vi "LVFunction_Imop_Compute_Strehl from HasoField.vi"(0 "HasoField.lvclass":refnum<class "HasoField.lvclass">, 5 "Path":path, 7 "defocus":sgl, 9 "param":T1={"flat_experimental_intensity"=TRUE, "flat_theoretical_intensity"=TRUE, "through_focus"=TRUE, "oversample"=TRUE}, 11 "error in (no error)":errorcluster) -> (4 "HasoField.lvclass dup":refnum<class "HasoField.lvclass">, 6 "strehl_ratio":sgl, 15 "error out":errorcluster)   [LabVIEW 2020]
doc: "Strehl ratio from Haso field function.\n\n--------------------------------------------------------------------------------\n\n<B>HasoFieldIn</B> : HasoField object.\n\n<B>HasoFieldOut</B> : HasoField object.\n\n<B>config_file_path</B> : Absolute path to the Haso configuration file.\n\n<B>flat_experimental_intensity</B> : Use flat experimental intensity.\n\n<B>flat_theoretical_intensity</B> : Use flat theoretical intensity.\n\n<B>through_focus</B> : Use through focus.\n\n<B>oversample</B> : Use oversample.\n\n<B>defocus</B> : Defocus parameter.\n\n<B>strehl_ratio</B> : Strehl ratio.\n\n<B>ErrorIn</B> : Error\n\n<B>ErrorOut</B> : Error"
uses:
  HasoField.lvclass
  LVClass_HasoField Read HasoField.vi
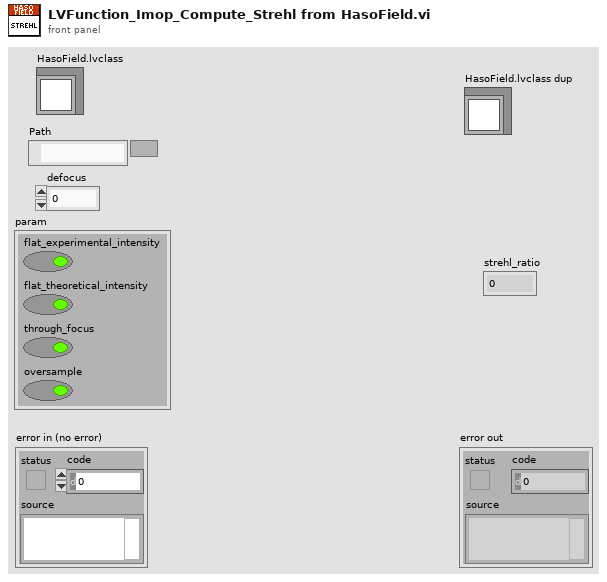
[diagram p1: front panel]
types:
  T1 = cluster{"flat_experimental_intensity":bool, "flat_theoretical_intensity":bool, "through_focus":bool, "oversample":bool}
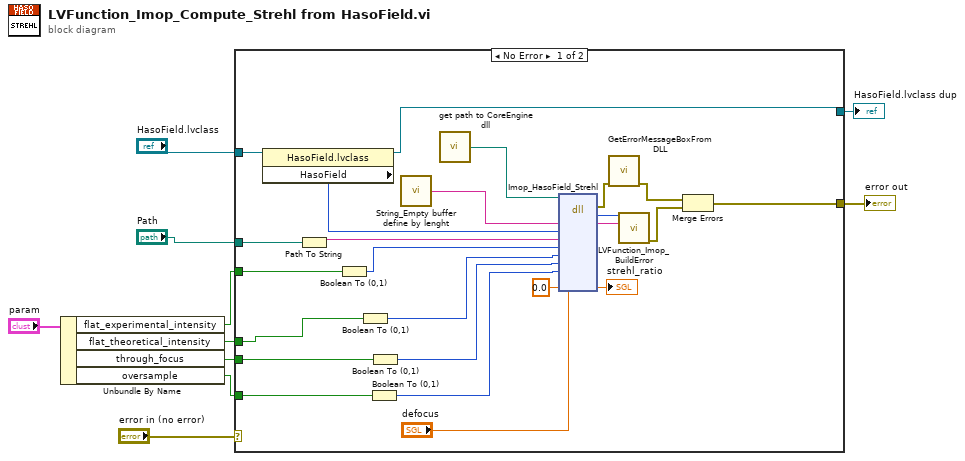
[diagram p0: block diagram]
diagram:
  n1 = Unbundle By Name("param") -> ("flat_experimental_intensity"=w5:bool, "flat_theoretical_intensity"=w4:bool, "through_focus"=w3:bool, "oversample"=w2:bool)
  n2 = case shown="No Error" "error in (no error)" {
    selector: "error in (no error)" -> [_ w36]
    tunnel: [w27 w36] -> w9
    tunnel: "Path" -> [w26 _]
    tunnel: "HasoField.lvclass" -> [w25 w35]
    tunnel: w5 -> [w15 _]
    tunnel: w4 -> [w14 _]
    tunnel: w3 -> [w13 _]
    tunnel: w2 -> [w12 _]
    tunnel: [w11 w35] -> w1
    frame No Error {
      n3 = property class="HasoField.lvclass"(reference=w25) -> (reference out=w11:refnum<class "HasoField.lvclass">, "HasoField"=w24:i32)  [unwired: 1 in, 1 out]
      n4 = Path To String(path=w26) -> (string=w23:string)
      n5 = Boolean To (0,1)(Boolean=w15) -> (0, 1=w20:i16)
      n6 = Boolean To (0,1)(Boolean=w14) -> (0, 1=w19:i16)
      n7 = Boolean To (0,1)(Boolean=w12) -> (0, 1=w17:i16)
      n8 = Boolean To (0,1)(Boolean=w13) -> (0, 1=w18:i16)
      n9 = call "String_Empty buffer define by lenght.vi"() -> ("Empty buffer"=w34:string)  [unwired: 1 in]
      n10 = call "get path to CoreEngine dll.vi"() -> ("path to c_interface_vc100.dll"=w31:path)  [unwired: 12 in, 3 out]
      n11 = dll-call lib="D:/2_trunk/Soft_haso/ImOpCoreEngine4_LV2011/DLLs/ImopEngine4_vc100.dll" fn="Imop_HasoField_Strehl"(path in=w31, "message"=w34, "hasoField"=w24, "config_file_path"=w23, "flat_experimental_intensity"=w20, "flat_theoretical_intensity"=w19, "through_focus"=w18, "oversample"=w17, "defocus"="defocus", "strehl_ratio"=sgl 0.0) -> (error out=w30:errorcluster, "return type"=w32:i32, "message"=w33:string, "strehl_ratio"=→"strehl_ratio":sgl)  [unwired: 9 in, 1 out]
      n12 = call "GetErrorMessageBoxFromDLL.vi"("error IN"=w30) -> ("error OUT"=w29:errorcluster)  [unwired: 10 in]
      n13 = call "LVFunction_Imop_BuildError.vi"("code"=w32, "String to Prepend to source (\"\")"=w33) -> ("error out"=w28:errorcluster)  [unwired: 13 in]
      n14 = Merge Errors(w29, w28) -> (w27:errorcluster)
    }
    frame Error {
    }
  }
  "error out" <- w9
  "HasoField.lvclass dup" <- w1
